vi "Destroy Enqueuer References.vi"(8 "error in (no error)":errorcluster, 11 "Requests":T1) -> (0 "error out":errorcluster)   [LabVIEW 2018, in "Scripting.lvlib" / "Actor.lvlib" / "Actor.lvclass"]
uses:
  Actor.lvclass
  Request-Enqueuers.ctl
  Get State.ctl
  State.ctl
  Stop.ctl
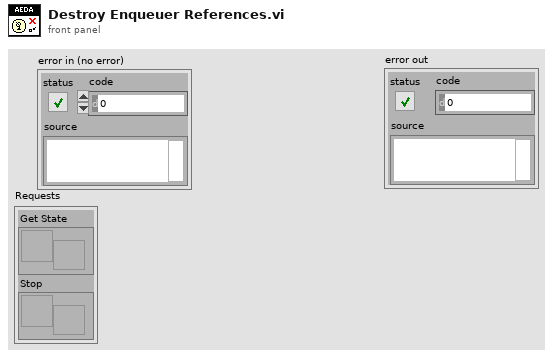
[diagram p1: front panel]
types:
  T1 = typedef "Scripting.lvlib/Actor.lvlib/Actor.lvclass/Request-Enqueuers.ctl" = cluster{"Get State":refnum<user-event>, "Stop":refnum<user-event>}
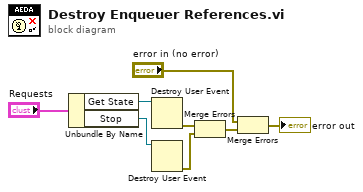
[diagram p0: block diagram]
diagram:
  n1 = Unbundle By Name("Requests") -> ("Get State"=w2:refnum<user-event>, "Stop"=w1:refnum<user-event>)
  n2 = Destroy User Event(user event=w2) -> (error out=w8:errorcluster)  [unwired: 1 in]
  n3 = Destroy User Event(user event=w1) -> (error out=w7:errorcluster)  [unwired: 1 in]
  n4 = Merge Errors(w8, w7) -> (w4:errorcluster)
  n5 = Merge Errors("error in (no error)", w4) -> (→"error out":errorcluster)
